vi "Utility Firmware Info.vi"(5 "Retry Attempts (0)":i32 min=0, 7 "Fast Comms (F)":bool, 8 "error in":errorcluster, 11 "VISA resource name":refnum<visa-resource-name>) -> (0 "error out":errorcluster, 1 "Firmware Version":string, 2 "Firmware Part Number":dbl, 3 "VISA resource name out":refnum<visa-resource-name>)   [LabVIEW 2020, in "ChromTech MX-Class Drivers.lvlib"]
doc: "Returns the firmware version and part number."
uses:
  <instrlib>/RxnRover/ChromtechNextGenDriver/ChromTech MX-Class Drivers.lvlib
panel:
  out "Response":string
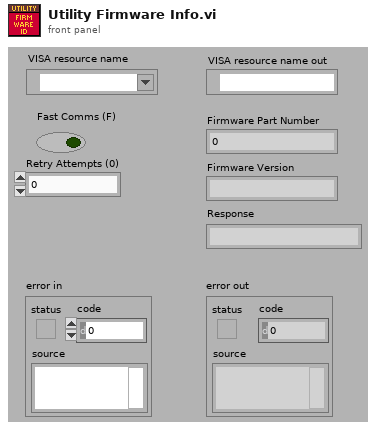
[diagram p1: front panel]
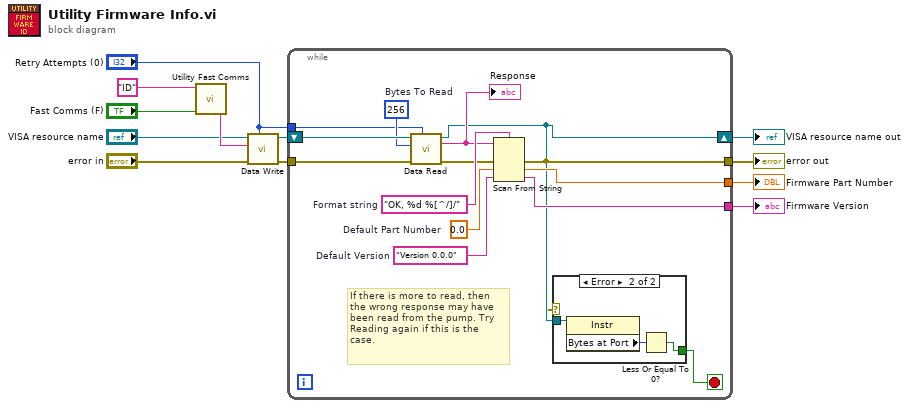
[diagram p0: block diagram]
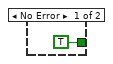
[diagram p2: hidden frame]
diagram:
  n1 = call <instrlib>:"Utility Fast Comms.vi"("Fast Comms"="Fast Comms (F)", "Command"="ID") -> ("Fast Command"=w11:string)  [unwired: 9 in]
  n2 = call <instrlib>:"Data Write.vi"("Retry Attempts (0)"="Retry Attempts (0)", "error in (no error)"="error in", "Command"=w11, "VISA Refnum in"="VISA resource name") -> ("error out"=w7:errorcluster, "VISA Refnum out"=w6:refnum<visa-resource-name>)  [unwired: 6 in]
  n3 = while {
    tunnel: [w25] -> w9
    tunnel: [w24] -> w8
    tunnel: "Retry Attempts (0)" -> [w16]
    shift-right: [w15] -> w2
    shift-left: w6 -> [w19]
    tunnel: w7 -> [w20]
    tunnel: [w14] -> w1
    stop <- w13 stop-if-true
    w18 = u32 256  # Bytes To Read
    w21 = "Version 0.0.0"  # Default Version
    w22 = 0.0  # Default Part Number
    w26 = "OK, %d %[^/]/"  # Format string
    # "If there is more to read, then\nthe wrong response may have\nbeen read from the pump. Try\nReading again if this is the\ncase."
    n4 = call <instrlib>:"Data Read.vi"("Retry Attempts (0)"=w16, "error in (no error)"=w20, "Bytes to read"=w18, "VISA Refnum in"=w19) -> ("error out"=w23:errorcluster, "read buffer"=w17:string, "VISA Refnum out"=w15:refnum<visa-resource-name>)  [unwired: 5 in]
    "Response" <- w17
    n5 = Scan From String(format string=w26, input string=w17, error in=w23, default 1=w22, default 2=w21) -> (error out=w14:errorcluster, output 1=w25:dbl, output 2=w24:string)  [unwired: 1 in, 2 out]
    n6 = case shown="Error" w14 {
      tunnel: w15 -> [_ w30]
      tunnel: [TRUE w28] -> w13
      frame No Error {
      }
      frame Error {
        n7 = property class="Instr"(reference=w30) -> ("Bytes at Port"=w29:u32)  [unwired: 1 in, 2 out]
        n8 = Less Or Equal To 0?(x=w29) -> (x <= 0?=w28:bool)
      }
    }
  }
  "VISA resource name out" <- w2
  "error out" <- w1
  "Firmware Part Number" <- w9
  "Firmware Version" <- w8
